vi "Write Default Values.vi"(10 "Default Values":T1[](array[typedef]), 11 "Toggle 6 in":refnum<class "Toggle 7.1.lvclass">) -> (3 "Toggle 6 out":refnum<class "Toggle 7.1.lvclass">)   [LabVIEW 2020, in "Toggle 7.1.lvclass"]
uses:
  Toggle 7.1.lvclass
  Controls/Register to Write.ctl
  Toggle 7.1.lvclass/Toggle 7.1.ctl
  PIC-device/PIC-Device.lvclass
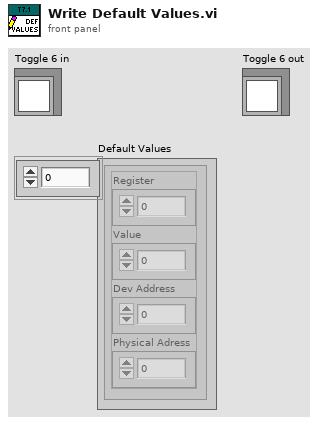
[diagram p1: front panel]
types:
  T1 = typedef "PIC-Device.lvclass/Register to Write.ctl" = cluster{"Register":u32, "Value":u32, "Dev Address":u32, "Physical Adress":u32}
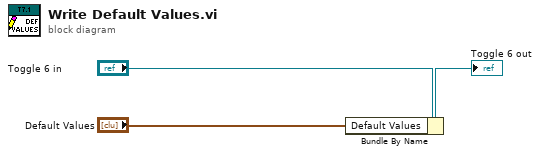
[diagram p0: block diagram]
diagram:
  n1 = Bundle By Name(cluster="Toggle 6 in", "Default Values"="Default Values") -> (→"Toggle 6 out":refnum<class "Toggle 7.1.lvclass">)
